vi "simx Get Object Group Data.vi"(0 "clientID":i32, 1 "objectType":i32, 2 "dataType":i32, 3 "handlesCount":i32, 4 "handles":i32, 5 "intDataCount":i32, 6 "intData":i32, 7 "error in (no error)":errorcluster, 8 "floatDataCount":i32, 9 "floatData":sgl, 10 "stringDataCount":i32, 11 "stringData":string, 12 "operationMode":i32) -> (16 "stringDataCount out":i32, 17 "stringData out":string, 18 "floatDataCount out":i32, 19 "floatData out":sgl, 20 "function return":i32, 23 "handlesCount out":i32, 24 "handles out":i32, 25 "intDataCount out":i32, 26 "intData out":i32, 27 "error out":errorcluster)   [LabVIEW 2019, in "PXL_V-REP.lvlib"]
doc: "EXTAPI_DLLEXPORT simxInt simxGetObjectGroupData(simxInt clientID,simxInt objectType,simxInt dataType,simxInt* handlesCount,simxInt** handles,simxInt* intDataCount,simxInt** intData,simxInt* floatDataCount,simxFloat** floatData,simxInt* stringDataCount,simxChar** stringData,simxInt operationMode);"
uses:
  PXL_V-REP.lvlib
  <userlib>/V-REP/remoteApi.dll
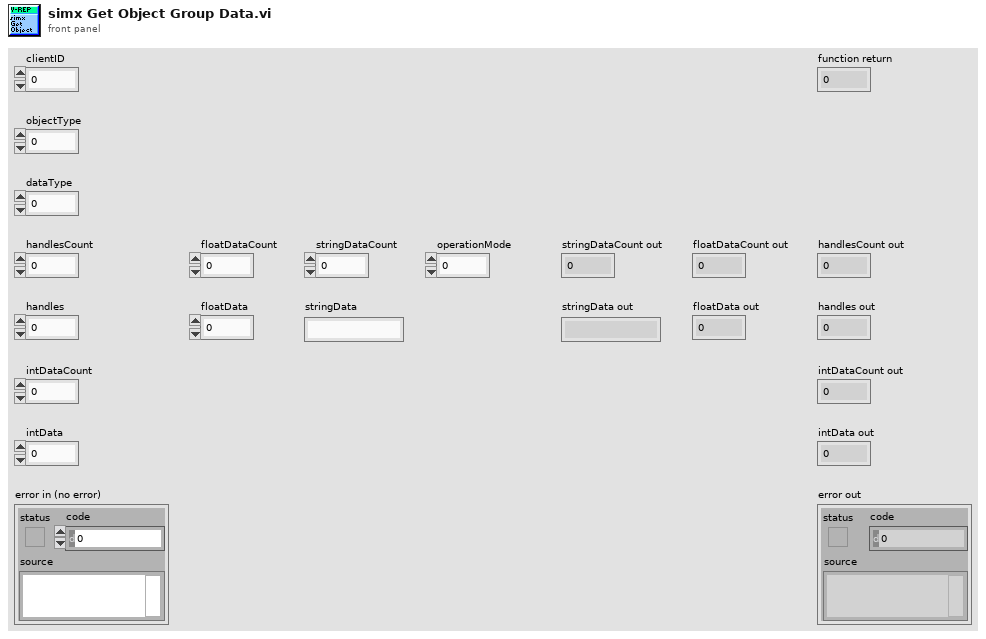
[diagram p1: front panel]
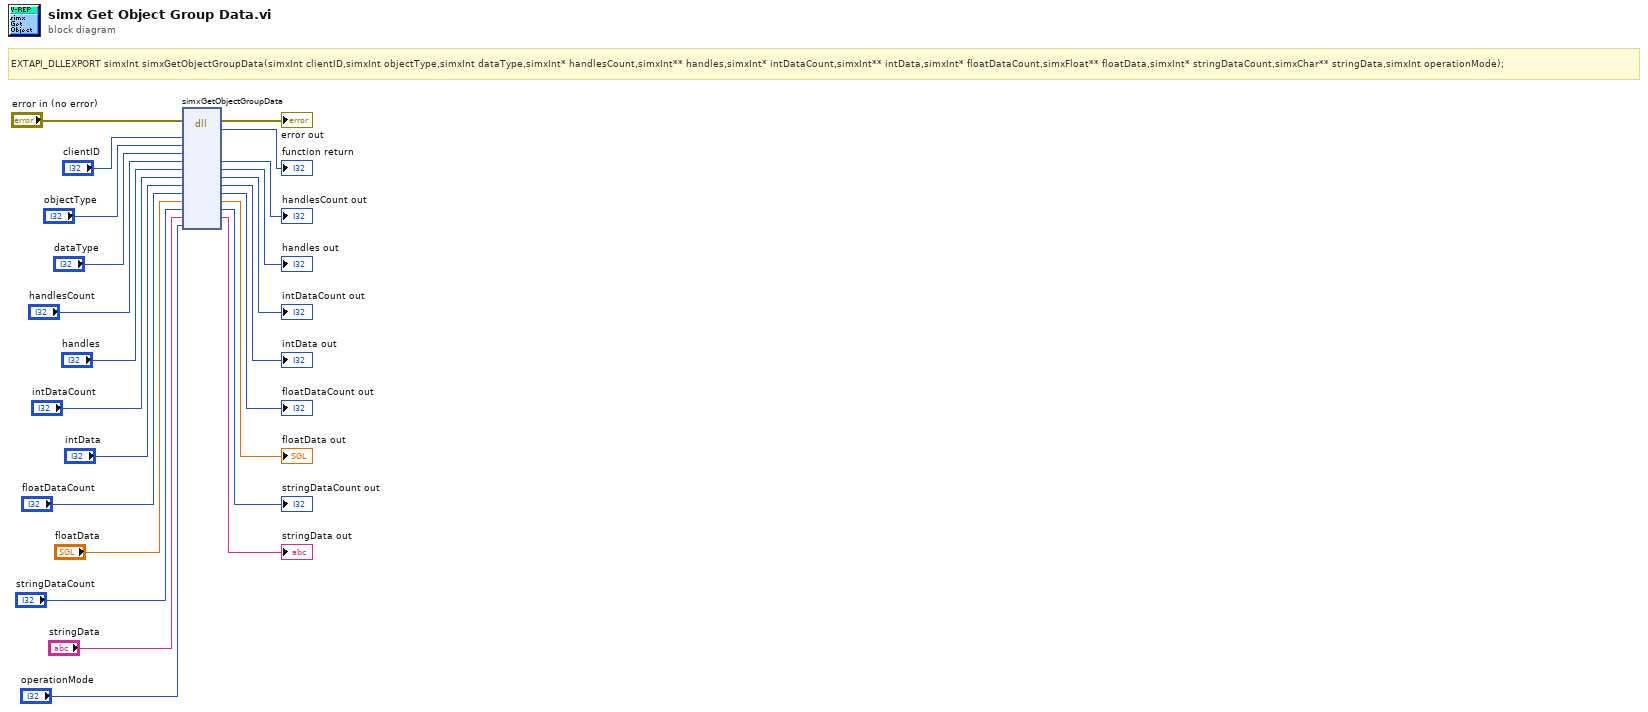
[diagram p0: block diagram]
diagram:
  # "EXTAPI_DLLEXPORT simxInt simxGetObjectGroupData(simxInt clientID,simxInt objectType,simxInt dataType,simxInt* handlesCount,simxInt** handles,simxInt* intDataCount,simxInt** intData,simxInt* floatDataCount,simxFloat** floatData,simxInt* stringDataCount,simxChar** stringData,simxInt operationMode);"
  n1 = dll-call lib="C:/Program Files (x86)/National Instruments/LabVIEW 2019/user.lib/V-REP/remoteApi.*" fn="simxGetObjectGroupData"(error in="error in (no error)", "clientID"="clientID", "objectType"="objectType", "dataType"="dataType", "handlesCount"="handlesCount", "handles"="handles", "intDataCount"="intDataCount", "intData"="intData", "floatDataCount"="floatDataCount", "floatData"="floatData", "stringDataCount"="stringDataCount", "stringData"="stringData", "operationMode"="operationMode") -> (error out=→"error out":errorcluster, →"function return":i32, "handlesCount"=→"handlesCount out":i32, "handles"=→"handles out":i32, "intDataCount"=→"intDataCount out":i32, "intData"=→"intData out":i32, "floatDataCount"=→"floatDataCount out":i32, "floatData"=→"floatData out":sgl, "stringDataCount"=→"stringDataCount out":i32, "stringData"=→"stringData out":string)  [unwired: 6 in, 1 out]
